vi "Save Start-up Configuration.vi"() -> ()   [LabVIEW 2016]
uses:
  Controllers/Application Controller/Start-up Configuration.ctl
  Controllers/Application Controller/Module Types.ctl
  <vilib>/Utility/config.llb/NI_LVConfig.lvlib
panel:
  in  "Detete old content":bool
  in  "File path":path
  in  "Initial Configuration":T1={"Load Modules"=[enum."Pulse Controller", enum."Monitor Controller", enum."NI-DAQmx", enum."NI-Scope", enum."Red Pitaya Digitizer", enum."VISA Device", enum."Red Pitaya Lockin", enum."Integrate Pulse", enum."Lockin Processor", enum."NHMFL Synthesizer"]}
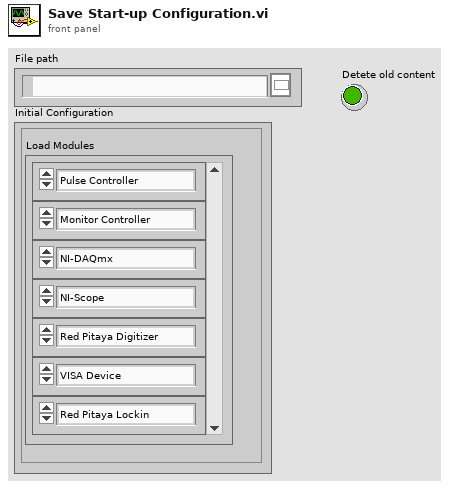
[diagram p1: front panel]
types:
  T1 = typedef "Start-up Configuration.ctl" = cluster{"Load Modules":T2[]}
  T2 = typedef "Module Types.ctl" = enum16{"NONE", "NI-DAQmx", "NI-Scope", "Red Pitaya Digitizer", "GaGe", "VISA Device", "Red Pitaya Lockin", "Monitor Controller", "Pulse Controller", "Integrate Pulse", "Lockin Processor", "File converter", "NHMFL Synthesizer", "Micron Hyperion", "Spectrum Recorder", "Resonance Detector", "TCP Communications", "Format Resonances"}
  T3 = typedef "NI_LVConfig.lvlib/Config Data RefNum.ctl" = refnum<k1>
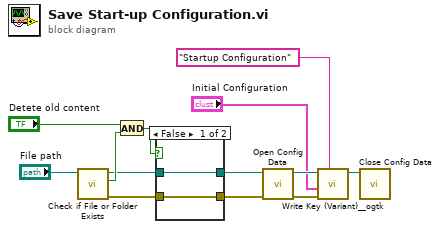
[diagram p0: block diagram]
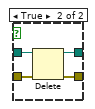
[diagram p2: hidden frame]
diagram:
  n1 = call <vilib>:"Check if File or Folder Exists.vi"("path"="File path") -> ("error out"=w3:errorcluster, "file or folder exists?"=w5:bool, "dup path"=w4:path)  [unwired: 8 in]
  n2 = And(x="Detete old content", y=w5) -> (x .and. y?=w6:bool)
  n3 = case shown="False" w6 {
    tunnel: w4 -> [w15 w19]
    tunnel: w3 -> [w14 w18]
    tunnel: [w15 w17] -> w2
    tunnel: [w14 w16] -> w1
    frame False {
    }
    frame True {
      n4 = Delete(path (use dialog)=w19, error in=w18) -> (deleted path=w17:path, error out=w16:errorcluster)  [unwired: 3 in, 1 out]
    }
  }
  n5 = call <vilib>:"Open Config Data.vi"("error in (no error)"=w1, "configuration file path"=w2) -> ("error out"=w12:errorcluster, "refnum"=w11:T3)  [unwired: 7 in, 1 out]
  n6 = call <userlib>:"Write Key (Variant)__ogtk.vi"("section"="Startup Configuration", "error in (no error)"=w12, "key-value"="Initial Configuration", "refnum"=w11) -> ("refnum out"=w13:T3)  [unwired: 6 in, 1 out]
  n7 = call <vilib>:"Close Config Data.vi"("refnum"=w13) -> ()  [unwired: 9 in, 2 out]
